vi "MathCad_Easy_Numeric_Get_Var.vi"(8 "error in (no error)":errorcluster, 10 "Variable  Name":string, 11 "Mathcad Reference":T1) -> (0 "error out":errorcluster, 2 "value":dbl format="%.2f", 3 "Mathcad Reference":T1)   [LabVIEW 2015]
doc: "Gets the numeric value in Mathcad. It gets the last definition of the variable.\n\nInputs\n Wrksht Ref--ActiveX Reference to Mathcad Worksheet Class\n Variable Name (string)- Name of the new variable to be retrieved.\nOutputs\n Wrksht Ref--ActiveX Reference to Mathcad Worksheet Class\n Value(Double)- Value of last definition of variable in worksheet."
uses:
  Mathcad Reference.ctl
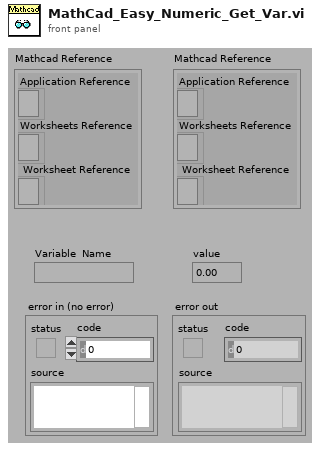
[diagram p1: front panel]
types:
  T1 = typedef "Mathcad Reference.ctl" = cluster{"Application Reference":refnum<k7>, "Worksheets Reference":refnum<k7>, " Worksheet Reference":refnum<k7>}
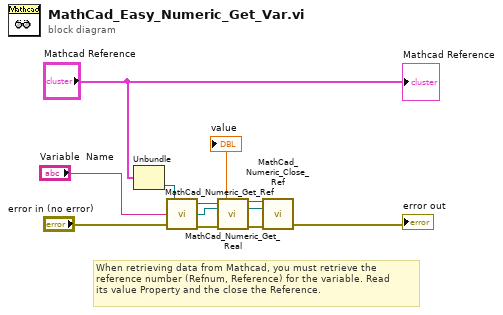
[diagram p0: block diagram]
diagram:
  # "When retrieving data from Mathcad, you must retrieve the \nreference number (Refnum, Reference) for the variable. Read \nits value Property and the close the Reference."
  n1 = Unbundle("Mathcad Reference") -> ("Worksheet Reference"=w1:refnum<k7>)  [unwired: 2 out]
  n2 = call "MathCad_Numeric_Get_Ref.vi"("error in (no error)"="error in (no error)", "Variable  Name"="Variable  Name", "Worksheet Reference In"=w1) -> ("error out"=w10:errorcluster, "Mathcad.INumericValue Refnum"=w4:refnum<k7>, "Worksheet Reference Out"=w12:refnum<k7>)
  n3 = call "MathCad_Numeric_Get_Real.vi"("Worksheet Reference In"=w12, "Mathcad.INumericValue Refnum In"=w4, "error in"=w10) -> ("value"=→"value":dbl, "Worksheet Reference Out"=w7:refnum<k7>, "Mathcad.INumericValue Refnum Out"=w6:refnum<k7>, "error out"=w5:errorcluster)  [unwired: 9 in]
  n4 = call "MathCad_Numeric_Close_Ref.vi"("error in"=w5, "Mathcad.INumericValue Reference"=w6, "IMathcadWorksheet Reference"=w7) -> ("error out"=→"error out":errorcluster)  [unwired: 2 in, 1 out]
  "Mathcad Reference" <- "Mathcad Reference"
